vi "未命名 3.vi"() -> ()   [LabVIEW 2018]
panel:
  out "数字":u8
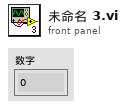
[diagram p1: front panel]
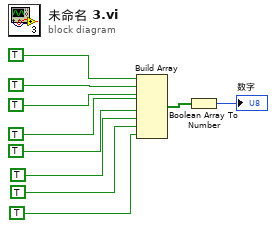
[diagram p0: block diagram]
diagram:
  n1 = Build Array(TRUE, TRUE, TRUE, TRUE, TRUE, TRUE, TRUE, TRUE) -> (w10:bool[])
  n2 = Boolean Array To Number(Boolean array=w10) -> (number=→"数字":u8)
